vi "Extract Bus Sections From Parameter List.vi"(0 "Parms List":string="*** BC ***\nMessage: Gun_One\nParameter: Data_01,8,0,8,1.0000,0.0000,0\nMessage: Gun_Two\nParameter: Data_02,8,0,8,1.0000,0.0000,0\nMessage: Get_It\nParameter: Data_00,1,0,8,1.0000,0.0000,0\n*** BM ***\nMessage: BM_05_T_04\nParameter: BM_Data_Parm_1,1,0,8,1.0000,0.0000,0\n*** RT ***\nMessage: RT_05_T_04_00\nParameter: RT Data T,1,0,8,1.0000,0.0000,0\nMessage: RT_0B_R_0A_00\nParameter: RT Data R,8,0,8,1.0000,0.0000,0\n\n") -> (4 "BC Section":string, 6 "BM Section":string, 8 "RT Section":string)   [LabVIEW 2013]
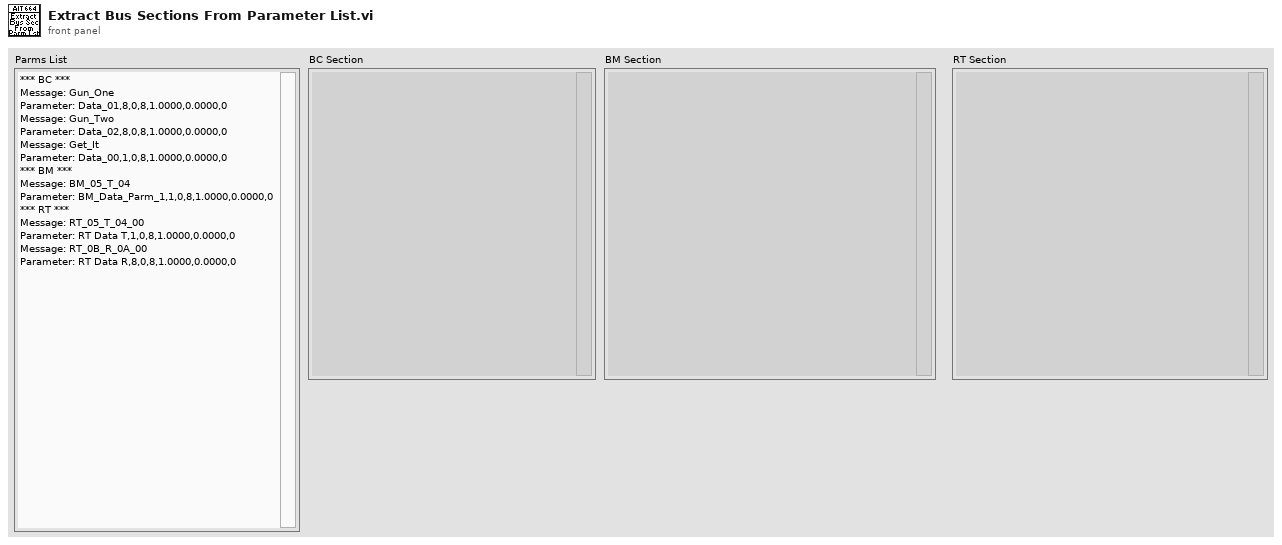
[diagram p1: front panel]
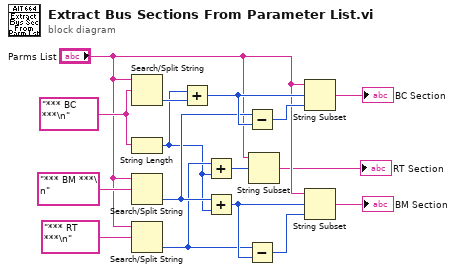
[diagram p0: block diagram]
diagram:
  w13 = "*** BC ***\n"
  n1 = Search/Split String(string="Parms List", search string/char (-)=w13) -> (offset of match=w14:i32)  [unwired: 1 in, 2 out]
  n2 = String Length(string=w13) -> (length=w5:i32)
  n3 = Search/Split String(string="Parms List", search string/char (-)="*** BM ***\n") -> (offset of match=w10:i32)  [unwired: 1 in, 2 out]
  n4 = Search/Split String(string="Parms List", search string/char (-)="*** RT ***\n") -> (offset of match=w6:i32)  [unwired: 1 in, 2 out]
  n5 = Add(x=w5, y=w14) -> (x+y=w12:i32)
  n6 = Add(x=w6, y=w5) -> (x+y=w3:i32)
  n7 = Add(x=w10, y=w5) -> (x+y=w8:i32)
  n8 = Subtract(x=w10, y=w12) -> (x-y=w11:i32)
  n9 = Subtract(x=w6, y=w8) -> (x-y=w9:i32)
  n10 = String Subset(string="Parms List", offset (0)=w3) -> (substring=→"RT Section":string)  [unwired: 1 in]
  n11 = String Subset(string="Parms List", offset (0)=w12, length (rest)=w11) -> (substring=→"BC Section":string)
  n12 = String Subset(string="Parms List", offset (0)=w8, length (rest)=w9) -> (substring=→"BM Section":string)
